vi "observacao.vi"() -> ()   [LabVIEW 2012]
uses:
  Control 1.ctl
  System.Windows.Forms
  Global_Telescopio.vi
  Global Tabs.vi
  Shared_160.lvlib
panel:
  out "timeStatShutterAlert":i32
  out "sendCommandShutter":bool
  out "shutterTimeOld":i32
  out "LEAF":i32
  in  "Default":string="DEFAULT"
  out "Flag ativo DEC":bool
  out "Flag ativo AH":bool
  out "Flag de erro p/ apagar lampada":bool
  out "Foco aux":dbl
  out "Cont-ShutOpen":timestamp
  out "Flag-ShutClose":bool
  out "Flag-ShutOpen":bool
  in  "erro lig":i32=3
  in  "erro des":i32=3
  in  "xxz":string
  out "Flag desligar":bool
  out "Flag ligar":bool
  out "Flag Stop":bool
  in  "AUX LAMPADA":bool
  out "Apontou":bool caption="Working Area"
  in  "AUX ABA":bool
  out "error out 5":errorcluster
  in  "error in (no error)":errorcluster
  out "AH_Destino":dbl format="%.9g"
  out "CONT DEC UTILS":i32
  out "CR DEC UTILS":i32
  out "CONT AH UTILS":i32
  out "CR AH UTILS":i32
  out "Erro PROTEC":i32=5
  out "Erro Lim":i32=5
  out "Flag Alarm":bool
  out "alarm Time":timestamp
  out "error out 4":errorcluster
  in  "Case Constant\n(See Context Help) 21":bool=TRUE
  in  "Case Constant\n(See Context Help) 20":bool=TRUE
  in  "Case Constant\n(See Context Help) 19":bool=TRUE
  in  "Case Constant\n(See Context Help) 18":bool
  in  "Case Constant\n(See Context Help) 17":bool=TRUE
  in  "Case Constant\n(See Context Help) 16":bool
  in  "LedPointing":bool=TRUE
  in  "Case Constant\n(See Context Help) 15":bool
  in  "Case Constant\n(See Context Help) 14":bool=TRUE
  in  "Case Constant\n(See Context Help) 13":bool=TRUE
  in  "Case Constant\n(See Context Help) 12":bool=TRUE
  in  "Case Constant\n(See Context Help) 11":bool
  in  "Case Constant\n(See Context Help) 10":bool
  in  "Case Constant\n(See Context Help) 9":bool
  in  "Disabled":u8=2
  in  "Case Constant\n(See Context Help) 8":bool=TRUE
  in  "Case Constant\n(See Context Help) 7":bool=TRUE
  in  "Case Constant\n(See Context Help) 6":bool
  in  "Case Constant\n(See Context Help) 5":bool
  in  "TRUE=HORA\nFALSE=GRAU":bool=TRUE
  in  "Case Constant\n(See Context Help) 4":bool
  in  "Case Constant\n(See Context Help) 3":bool
  in  "Case Constant\n(See Context Help) 2":bool
  in  "Case Constant\n(See Context Help)":bool
  out "TA3":u32
  out "TA2":u32
  out "TF2":u32
  out "TF1":u32
  out "TA1":u32
  out "Tick Cupula":u32
  out "T2 3":u32
  in  "ESTADO ABRIR":string
  in  "ESTADO FECHAR":string
  out "T2 2":u32
  out "T1 2":u32
  out "T2":u32
  out "T1":u32
  out "DEC":string="00 00 00,00"
  out "Hour Angle 2":string="00 00 0,00" caption="AH"
  in  "TIMER TICK":u32
  in  "STOP":bool
  in  "News":bool
  out "AtmosferaStr":string
  in  "BtShutterClose":bool caption="DOME SHUTTER"
  out "HA obs":dbl
  out "Time to Limit":string
  in  "Clear All Messages":bool
  out "FiltroDuplo":bool
  out "ObjCentrado":bool
  out "Timeout PROT":u32
  out "LIMITE":bool
  in  "DestCUP":i16
  in  "DestAH":dbl
  in  "DestDEC":dbl
  in  "M_CUP":i32
  out "TimeoutCUP 2":u32
  out "TimeoutAH 2":u32
  out "TimeoutDEC 2":u32
  in  "Max":dbl=2300.0
  in  "Min":dbl=200.0
  out "error out":errorcluster
  out "TUBO_STAT":string
  out "CUP_STAT":string
  out "DEC_STAT":string
  out "AH_STAT":string
  out "FOCO_ENC":string
  out "DEC_ENC":string
  out "AH_ENC":string
  out "RA on Target":bool
  in  "BtOnTatget":bool
  out "Offset DEC":dbl format="%#.2f"
  out "Offset RA":dbl format="%#.2f"
  out "Mount Fine Movement":bool
  out "Mount Gross Movement":bool
  in  "follow redirects (T)":bool=TRUE
  out "header":string
  out "subarray":string[][](array[string])
  out "Draw Area 4":cluster{"Width":u32, "Height":u32}
  out "Draw Area 3":cluster{"Width":u32, "Height":u32}
  in  "sair":bool
  out "Saida Path string":string
  out "AUX EDITA RA":string caption="Name"
  out "Sideral time":string caption="ST"
  out "UT":string
  out "FLAG SET COORD":bool
  out "AUX EDITA PMDEC":string caption="Name"
  out "AUX EDITA PMRA":string caption="Name"
  out "AUX EDITA EPOCH":string caption="Name"
  out "AUX EDITA DEC":string caption="Name"
  out "AUX EDITA Name":string caption="Name"
  out "Hour Angle":string="00 00 0,00"
  in  "DECTARGET":string
  in  "AHTARGET":string
  out "Zenital angle":dbl
  out "SlideEnviromental":dbl(slide) caption="Progress ..." scale=0.0..100.0
  out "RA AUX":string
  out "EPOCH AUX":string
  out "Draw Area 2":cluster{"Width":u32, "Height":u32}
  out "SYSTEM MESSAGES":string
  out "Data Acquisition Activity":bool
  out "Auto guider Activity":bool
  out "Security Zone":bool
  out "Precess Data out-of-date":bool
  out "D...":bool
  out "C...":bool
  out "B...":bool
  out "A...":bool
  out "DEC on Target":bool
  out "Dome on Target":bool
  out "Remote User in Control":bool
  out "Air Mass":dbl
  out "Epoch":dbl
  out "Right Ascention":string="00 00 00,00"
  out "Declination":string="00 00 00,00"
  out "Azimuth":dbl
  out "Wind Chill":dbl
  out "Boolean 11":bool
  out "Wind Dir":string
  in  "Int/Ext":bool=TRUE
  out "Temperature":dbl
  out "Humidity":dbl
  out "Dew Point":dbl
  out "Wind Speed":dbl
  out "Pressure":dbl
  in  "RESTART METEOR":bool
  in  "VARIABLE \nTRACKING":bool
  out "LED VAR TRACKING":bool
  out "LED GUIDER":bool
  out "Led Chave Dome":bool
  out "LED MOUNT":bool
  in  "GUIDER":bool
  in  "DOME":bool
  in  "MOUNT":bool
  out "NAME":string
  out "DEC":string
  out "RA":string
  in  "Tab Control":T1(tab)=enum."Test Only"
  in  "IMAGE 5":bool
  out "Image":picture
  in  "PictureBox":refnum<k24>(container)
  out "Image 2":picture
  in  "IMAGE 2":bool
  out "error out 3":errorcluster
  out "error out 2":errorcluster
  in  "IMAGE 4":bool
  out "Image 4":picture
  out "pressão atm":string
  out "hum local":string
  out "Temp amb":string
  in  "IMAGE 3":bool
  out "Image 3":picture
  in  "IMAGE 6":bool
  out "Image 3a":picture
  out "C. AH":i32
  out "DOMO_ENC":string
  out "Proteção":bool
  in  "M_PROT":i32
  out "dt":u32
  out "TUBO":bool[](array[boolean])
  out "CUP":bool[](array[boolean])
  out "DEC":bool[](array[boolean])
  out "RA":bool[](array[boolean])
  in  "statCUP":i32
  in  "statAH":i32
  in  "statDEC":i32
  out "statCUP 2":i32
  out "TimeoutCUP":u32
  out "Azimute cup":u16
  out "PosCUP":i16
  out "dtAUX2":u32
  out "dtAUX3":u32
  in  "Phx":dbl=200.0 caption="Setpoint" min=200.0 max=2300.0 step=1.0
  out "PosAH":dbl
  out "PosDEC":dbl
  out "dec=":bool
  out "ah=":bool
  in  "CR AH":i32
  in  "CR DEC":i32
  out "C. DEC":i32
  in  "M_AH":i32
  in  "M_DEC":i32
  in  "Stop All":bool
  in  "Setup, Pointing & Guiding":T2(tab)=enum."POINTING"
  in  "RA Max 2":i32 min=-6 max=23
  in  "RA Min 2":i32 min=-6 max=23
  out "Erro":bool
  in  "MAG Max":dbl min=-9.0 max=100.0
  in  "MAG Min":dbl min=-9.0 max=25.0
  in  "DEC Max":i32 min=-90 max=90
  in  "DEC Min":i32 min=-90 max=90
  in  "RA Max":i32 caption="AH Max" min=-6 max=23
  in  "RA Min":i32 caption="AH Min" min=-6 max=23
  in  "Filter RA":bool
  in  "Slide old":i32
  out "Tot Linhas":i32
  in  "Open BSC":bool
  in  "Slide":dbl(slide) min=0.0 max=24.0 step=0.024 scale format="%#_3g"
  in  "EDIT":bool
  in  "Insert":bool
  out "List File":string
  in  "Upload":bool
  in  "Open":bool
  in  "Save AS":bool
  in  "Save":bool
  in  "Clear ALL":bool
  in  "SET coord":bool
  in  "Delete":bool
  in  "Multicolumn Listbox":i32[](listbox)
  out "ScaleMin":string
  out "ScaleMax":string
  out "DEC obs":dbl format="%.9f"
  out "RA obs":dbl format="%.9f"
  in  "ChkPointPrecessed":bool
  in  "Processa Centragem":bool
  out "PM_DEC":string
  out "PM_RA":string
  out "LedPointing":bool caption="Telescope Pointing"
  out "TimeoutAH":u32
  out "TimeoutDEC":u32
  out "AtualDEC":dbl format="%.9f"
  out "MeanDEC":string
  out "MeanRA":string
  in  "MAG":string
  out "Zenital Angle":string
  out "Air Mass":string
  out "Tempo Obs":string
  in  "BtPointPrecess":bool
  in  "ChkCalGlobal":bool=TRUE
  in  "ChkCalLocal":bool caption="Use Local Zero"
  in  "ChkPoinLampOFF":bool=TRUE
  in  "ChkPointRNA":bool
  in  "ChkModel":bool=TRUE
  in  "ChkWindDown":bool
  in  "ChkOpenShutter":bool
  in  "ChkDomeEnable":bool
  out "LedPointWorkArea":bool caption="Working Area"
  in  "BtTargetPoint":bool
  out "StrPointTargetDEC":string caption="Declination"
  out "StrPointTargetRA":string caption="Right Ascension"
  in  "BtPointObjClear":bool
  in  "StrPointObjPMDEC":string caption="DEC Proper Motion"
  in  "StrPointObjPMRA":string caption="RA Proper Motion"
  in  "StrPointObjName":string caption="Name"
  in  "StrPointObjEpoch":string caption="Epoch"
  in  "StrPointObjDEC":string caption="Declination"
  in  "StrPointObjRA":string caption="Right Ascension"
  out "MOV_IDX_DEC":bool
  out "MOV_IDX_AH":bool
  out "LatchDeslocDEC":dbl caption="DEC"
  out "LatchDeslocRA":dbl caption="RA"
  in  "ClearDeslocDEC":bool
  in  "ClearDeslocRA":bool
  out "DeslocDEC":dbl caption="DEC" format="%#.1f"
  out "DeslocRA":dbl caption="RA" format="%#.1f"
  in  "Delete Calagem":bool
  in  "Global":bool caption="Local"
  in  "Calagem":bool
  in  "Up HS":bool
  in  "Right HS":bool
  in  "Down HS":bool
  in  "Left HS":bool
  in  "Velocity (arcsec/sec)":i32(slide) min=0 max=600 scale=0.0..600.0
  in  "BtPrecGO":bool
  in  "BtPrecCentrar":bool
  in  "PreciseOffsetDEC":dbl caption="DEC" min=-10000.0 max=10000.0 step=1.0 format="%.3g"
  in  "PreciseOffsetRA":dbl caption="RA . cos(delta)" min=-10000.0 max=10000.0 step=1.0 format="%.3g"
  in  "Habilita Movimento":bool=TRUE
  in  "Y STAR":i32=1 min=1 max=400 step=1
  in  "X STAR":i32=1 min=1 max=400 step=1
  in  "XY CENTER":bool
  in  "Y CENTER":i32=1 min=1 max=400 step=1
  in  "X CENTER":i32=1 min=1 max=400 step=1
  in  "ClearRA":bool
  in  "ClearDEC":bool
  in  "DEC RATE":i32 min=-2000 max=2000 step=1
  in  "RA  RATE":i32 min=-2000 max=2000 step=1
  out "x+y":timestamp
  in  "plus":bool
  in  "minus":bool
  in  "SetDefaultFocus":bool
  out "On Position":bool
  out "Foco":dbl(slide) scale=200.0..2300.0
  in  "Setpoint":dbl=200.0 min=200.0 max=2300.0 step=1.0
  in  "GO":bool
  in  "Focus +":bool
  in  "Focus -":bool
  in  "New Angle":string="    0.0"
  out "Default Angle":string="      0.00"
  in  "SetRotatorDefAngle":bool
  in  "Set Rotator Angle":bool
  out "Rotator Angle":string="  0.00" caption="for  GUIDING"
  out "StatShutterFile":string
  out "Command":string
  in  "CCW":bool
  out "RefreshShutterState":bool
  in  "BtParavStop":bool
  in  "BtParavUp":bool
  in  "BtParavDown":bool
  out "LedShutter":bool
  out "TimeoutTrap":u32
  out "StatShutter":string caption="Control State"
  in  "BtShutClose":bool
  in  "BtShutOpen":bool
  out "StatDome":string caption="Control State"
  in  "BtDomeSTOP":bool
  in  "BtDomeGO":bool caption="DOME"
  in  "DomeNewPos":i32=30 caption="New Position" min=0 max=360
  out "PosCup":i16 caption="Position"
  in  "CW":bool
  out "LED ACTION":bool
  out "LED MODE":bool
  in  "ACTION":bool
  in  "MODE":bool
  in  "Default Met":bool=TRUE
  in  "PROTEÇÃO":bool
  in  "STOP":bool
  in  "Enable Centragem":bool=TRUE
  in  "GO":bool
  in  "StrPointObjDEC 2":string caption="DEC"
  in  "StrPointObjRA 2":string caption="AH"
  out "MOVING":bool
  in  "FLAT-FIELD":bool
  in  "BtUtilPark":bool
  in  "ECASS":bool
  in  "BtUtilZenith":bool
  in  "TabInstrumento":T3(tab)=enum."Cam 1"
  out "Posição Rede":i32=10 caption="Largura da Fenda" min=10 max=5000 step=1
  in  "HomePrisma":T4 caption="DOME"
  in  "HomeEspelho":T4 caption="DOME"
  in  "HomeFenda":T4 caption="DOME"
  in  "IronArc":bool=TRUE
  out "Boolean":bool
  out "Largura da Fenda 2":dbl=10.0 caption="Largura da Fenda" min=10.0 max=5000.0 step=1.0
  in  "Prisma das Lâmpadas":bool
  out "Position":string
  in  "Largura da Fenda":dbl=10.0 min=10.0 max=5000.0 step=1.0
  in  "Go Largura da Fenda":bool caption="DOME"
  in  "Angulo da rede de difração":i32=10 caption="Ângulo da Rede" min=10 max=99989 step=1
  in  "Go Angulo de Difração":bool caption="DOME"
  in  "Incand":bool=TRUE
  in  "Neon":bool=TRUE
  in  "Cathode":bool=TRUE
  out "Ang. Fenda":dbl
  in  "Go_Coudé":bool
  in  "Radio Buttons":enum32{"Azul", "Visível", "Vermelho"}(radio)
  out "EndTime":u32
  out "ledAzul":bool
  out "ledVisivel":bool
  out "ledVermelho":bool
  in  "MENSAGEM":string="EM MOVIMENTO"
  out "MENSAGEM 2":string="EM MOVIMENTO"
  out "#2":bool
  out "#3":bool
  out "#4":bool
  out "PosSecundario":bool
  out "Cjto_3":bool
  out "EspAtual":string
  out "parou":bool
  out "parou 2":bool
  out "Posição Espelho":dbl=10.0 caption="Largura da Fenda" min=10.0 max=5000.0 step=1.0
  out "parou 3":bool
  out "Output Message":string
  in  "stopEcass":bool
  out "SlideEcass":u8(slide) caption="Espelho movendo..." max=100 scale=0.0..100.0
  out "LedRep":bool
  out "LedCal":bool
  in  "Sent_EspLampCass":bool
  out "LedHe":bool
  out "LedNe":bool
  in  "He-Ar":bool
  in  "Ne":bool
  in  "stopCam1":bool
  out "SlideCam1":u8(slide) caption="Espelho movendo..." max=100 scale=0.0..100.0
  out "LedRepCam1":bool
  out "LedCalCam1":bool
  in  "Sent_EspDesvFeixe":bool
  in  "Go_filtro":bool
  in  "Filtro":string(combo)
  in  "Mover/Parar":bool
  out "Recuar":bool
  in  "Sentido":bool=TRUE
  in  "Velocidade":bool
  out "Rapido":bool
  out "Lento":bool
  out "Avancar":bool
  out "Comando":string
  in  "Mensage Alarme":string="To light up close the Shutter !"
  out "CoudeSel":bool
  in  "Coude":bool
  in  "BtCalFlatField":bool
  in  "ChkCalLamp4":bool
  in  "ChkCalLamp3":bool
  in  "ChkCalLamp2":bool
  in  "ChkCalLamp1":bool
  in  "BtCalTurnOff":bool
  in  "BtCalTurnOn":bool
  out "StrongSel":bool
  out "MediumSel":bool
  out "WeakSel":bool
  in  "Strong":bool
  in  "Medium":bool
  in  "Weak":bool
  # "TELESCOPE CONTROL SYSTEM\nPICO DOS DIAS OBSERVATORY"
  # "Status Information"
  # "System Positions"
  # "Environmental Status"
  # "EXT"
  # "INT"
  # "mBar"
  # "o"
  # "C"
  # "Km/h"
  # "%"
  # "o"
  # "o"
  # "C"
  # "C"
  # "CLOUSURE LIMITS"
  # "Wind Speed            >  70 Km/h\nRelative Humidity    >  97 %\nInternal Dewpoint  <  0.5  C\nExternal Dewpoint <  1.0  C"
  # "OBJECT"
  # "TRACKING ENABLE"
  # "Conector 4"
  # "Conector 3"
  # "ALARME\nATENÇÃO\nERROS\nOCUPADO"
  # "Proteção\n\nTracking\nVar_Track"
  # "Rapido\nLigeiro\nFino\nRun"
  # "Motor\nIDX_Rdy\nManual"
  # "BSC FILTERS"
  # "LIST FILE"
  # "OBJECT INPUT"
  # "TARGET"
  # "OPTIONS"
  # "MANUAL OFFSET"
  # "PRECISE OFFSET"
  # "N"
  # "E"
  # "W"
  # "arcsec"
  # "arcsec"
  # "S"
  # "DISPLACEMENT"
  # "CALAGEM"
  # "PODE NÃO FUNCIONAR CORRETAMENTE!"
  # "STAR CENTERING"
  # "VAR. TRACKING"
  # "AUTO-GUIDER COORDINATES"
  # "1) Entrar X e Y do cursor do Autoguider correspondente à posição de centragem nas entradas X CENTER e Y CENTER. \n2) Após apontamento, entrar em X STAR e Y STAR os valores de X e Y do Autoguider com o \"Guide Box\" sobre o objeto apontado. \n3) Clicar em MOVE STAR TO CENTER."
  # "Focus Position"
  # "(instrument)"
  # "Continuous Movement"
  # "Fine Tuning"
  # "ATENÇÃO:\nO Rotator ainda não está integrado ao sistema de controle e como sua posição afeta a guiagem, sempre que o rotator for girado manualmente é necessário digitar o valor de sua nova posição no controle \"New Angle\" e pressionar \"SET NEW\".\n\nPressionar \"SET NEW\" ou \"SET DEFAULT\" não gira o rotator!"
  # "ROTATION"
  # "SHUTTER"
  # "WINDSCREEN"
  # "Covers"
  # "FIXED POSITIONS"
  # "Acquisition System\nON TARGET command"
  # "Select one Mirrror"
  # "Mirror #2"
  # "Mirror #3"
  # "Mirrors Drivers"
  # "Lâmpadas de Calibração"
  # "Espelho das Lâmpadas de Calibração"
  # "Posição"
  # "Repouso"
  # "Ativo"
  # "LIGA"
  # "LIGA"
  # "DESL."
  # "DESL."
  # "Espelho do Eucalyptus"
  # "Roda de filtros"
  # "Posição"
  # "Repouso"
  # "Ativo"
  # "Espelho de Campo"
  # "Recuar"
  # "Avançar"
  # "Rápido"
  # "Lento"
  # "CALIBRATION LAMPS"
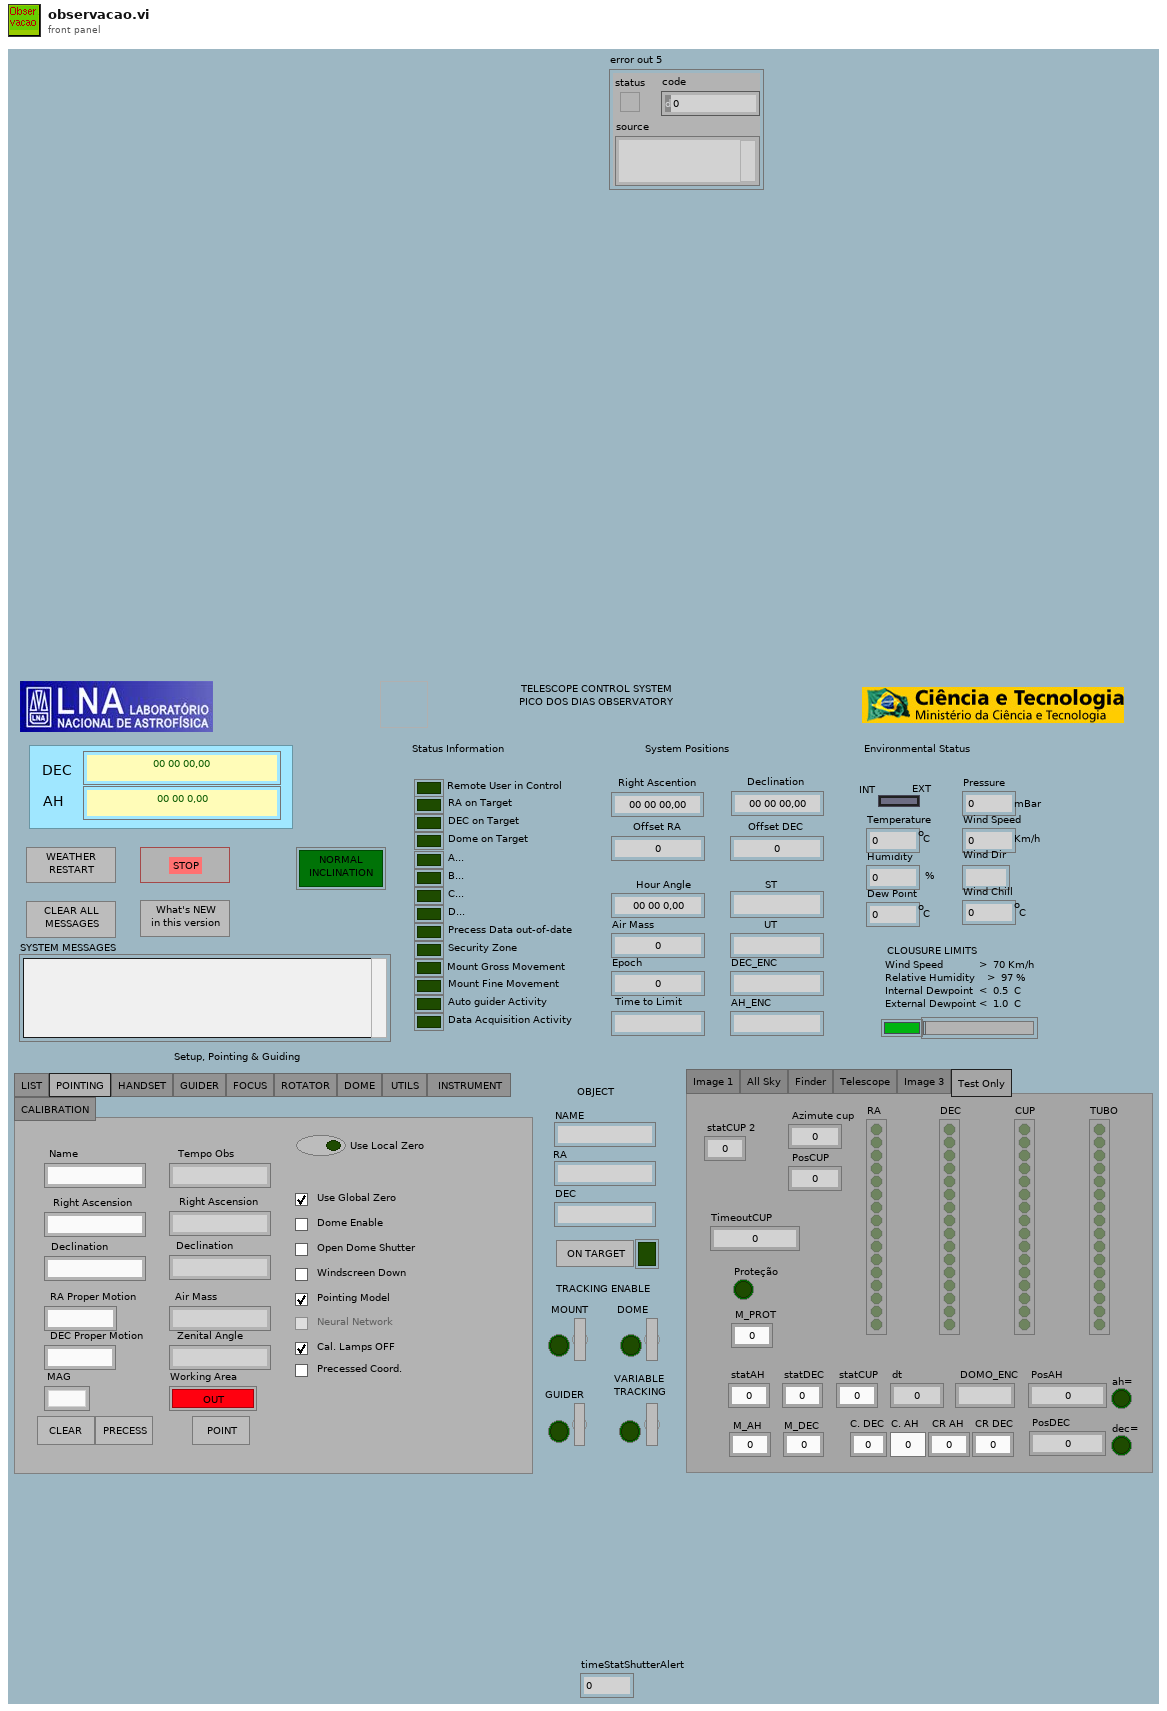
[diagram p1: front panel]
types:
  T1 = enum32{"Image 1", "All Sky", "Finder", "Telescope", "Image 3", "Test Only"}
  T2 = enum32{"LIST", "POINTING", "HANDSET", "GUIDER", "FOCUS", "ROTATOR", "DOME", "UTILS ", " INSTRUMENT ", "CALIBRATION"}
  T3 = enum32{"Coude", "Casseg.", "Eucalyp.", "Cam 1", "Cam 2", "Cam IV.", "Polarim.", "Fotrap"}
  T4 = typedef "Control 1.ctl" = bool
  T5 = enum32{"Page Enabled", "Page Disabled", "Page Disabled & Grayed"}
  T6 = enum16{"open", "replace", "create", "open or create", "replace or create", "replace or create with confirmation"}
  T7 = enum16{"open", "open or create", "create or replace", "create"}
  T8 = enum16{"open", "open or create", "create or replace", "create", "open (read only)"}
  T9 = typedef "LVRemotePanelConnectionsTypeDef.ctl" = cluster{"VI Name":string, "Remote":string, "UserName":string, "Port":i32, "Status":enum32{"Viewing", "Waiting For Control", "Controlling"}, "Create Time":timestamp, "Status Time":timestamp, "Control End Time":timestamp}[]
  T10 = enum8{"Enabled", "Disabled", "Disabled and Grayed Out"}
  T11 = cluster{"left":i16, "top":i16, "right":i16, "bottom":i16}
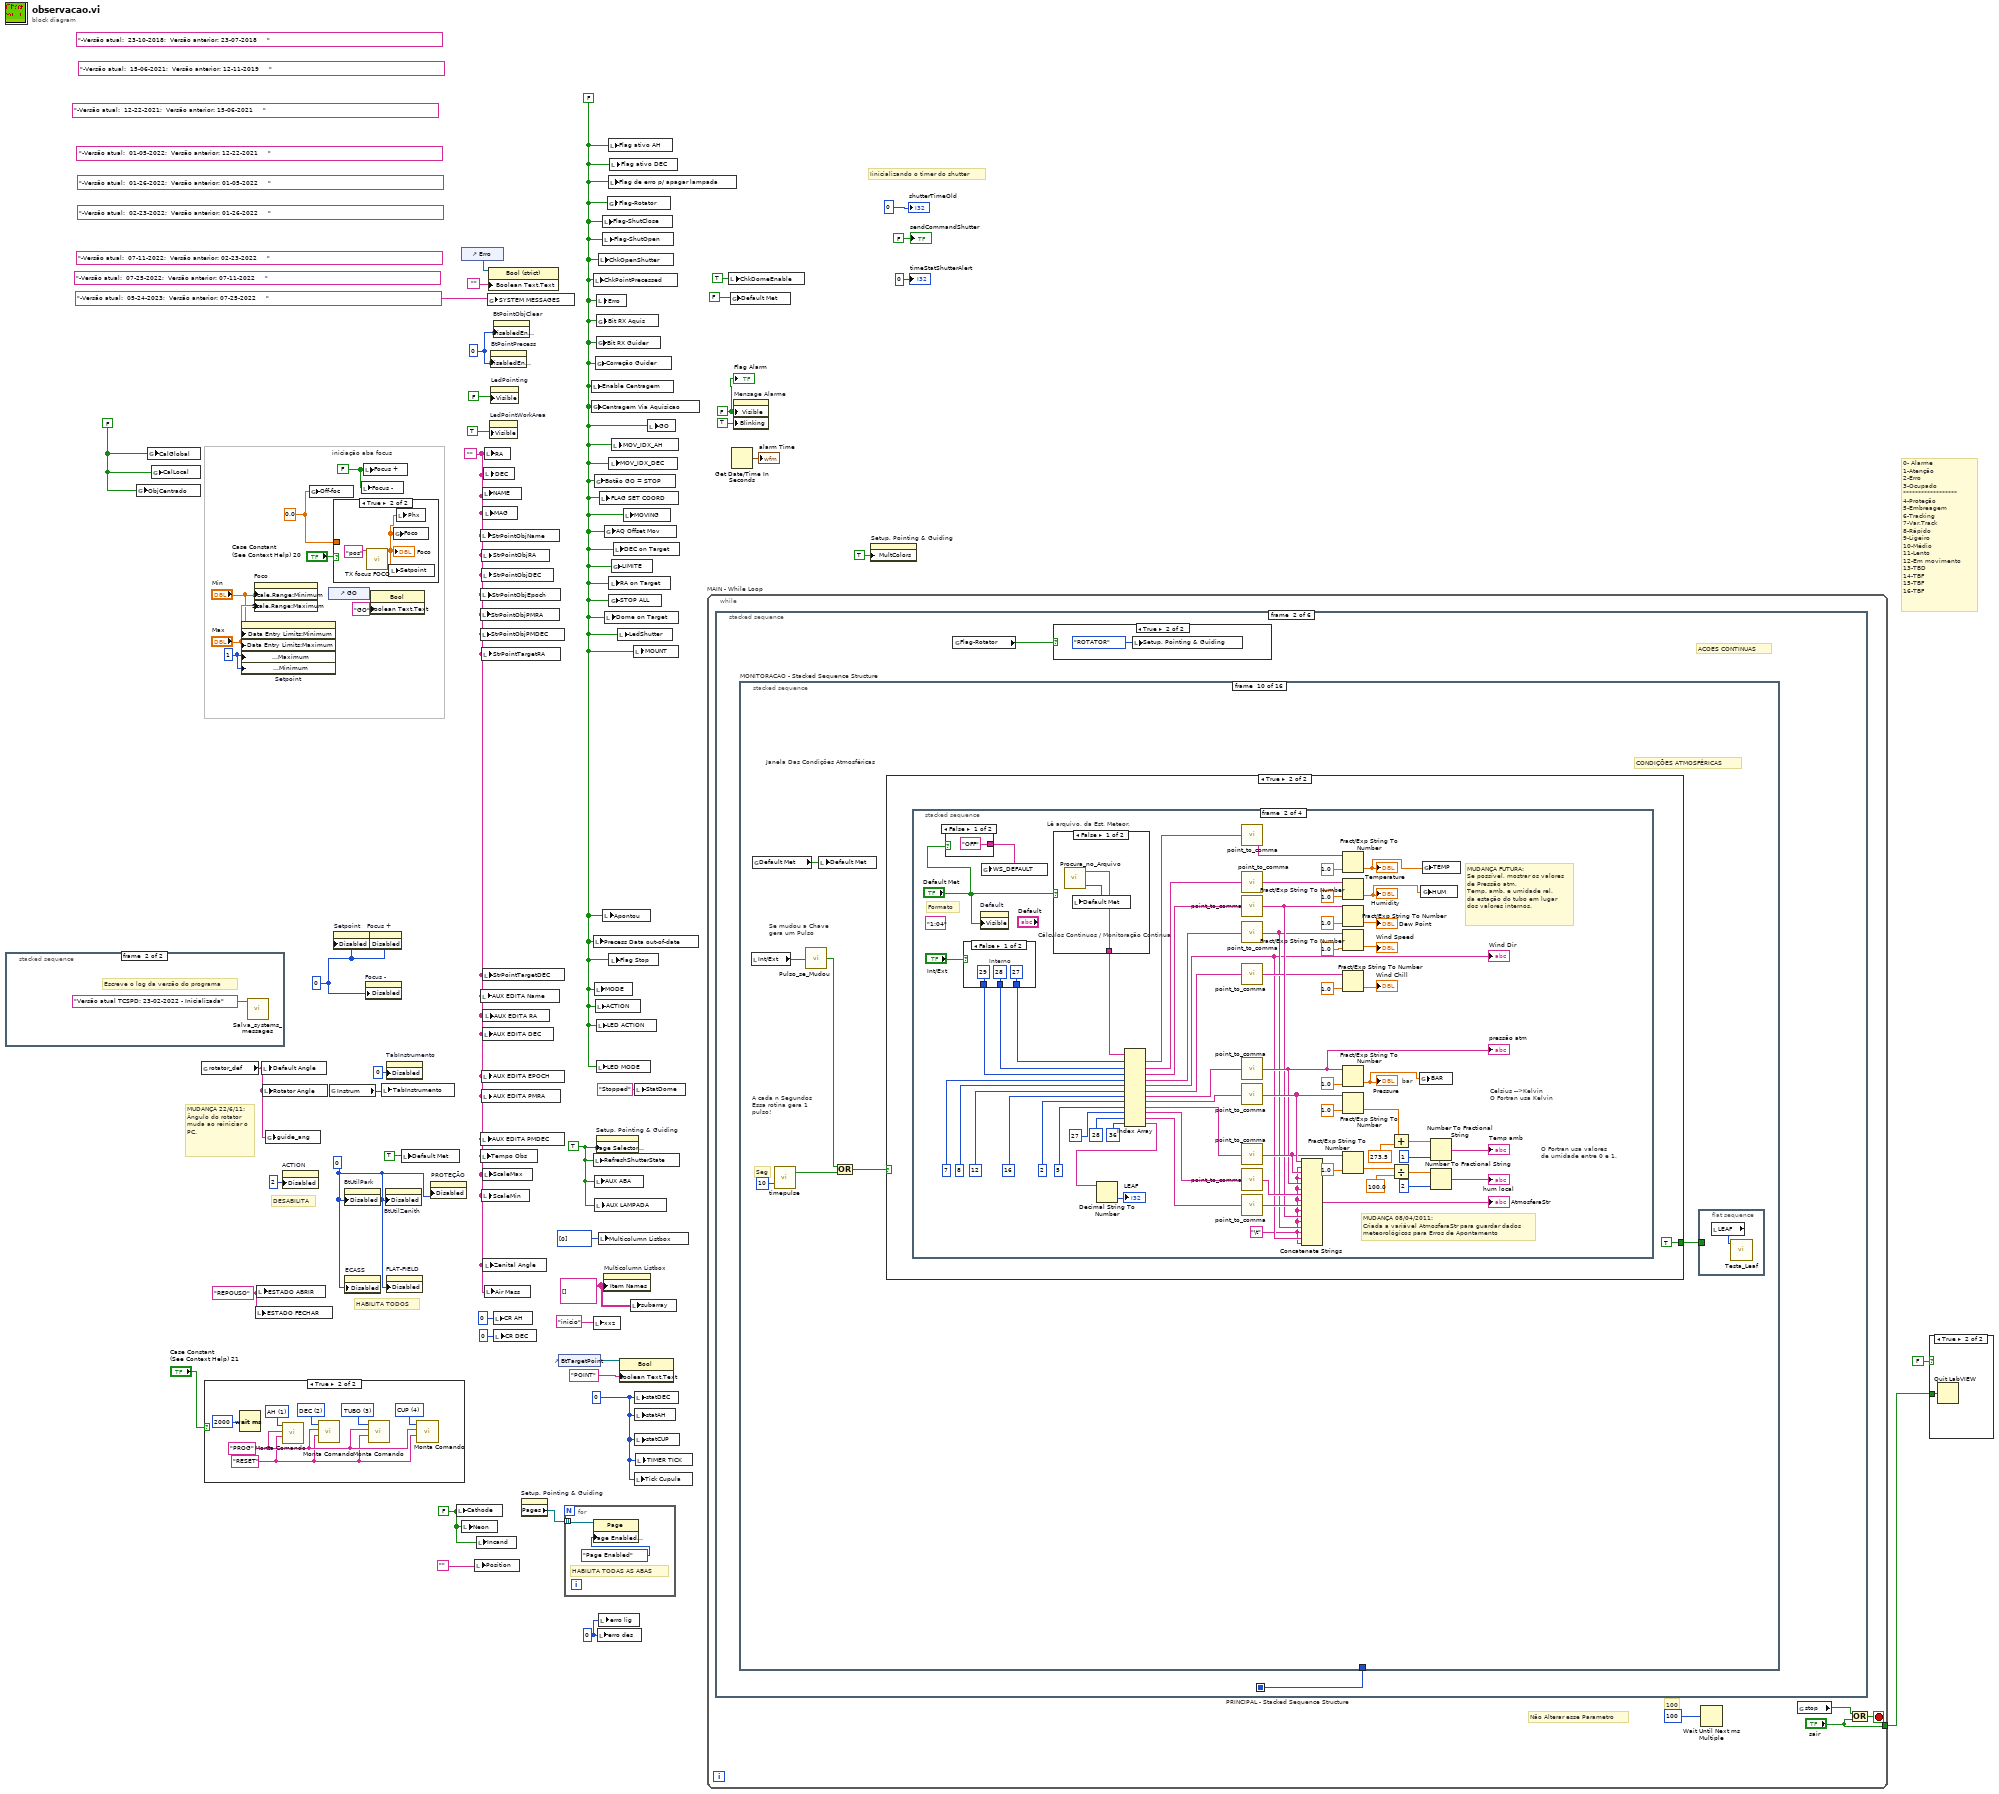
[diagram p0: block diagram]
diagram:
  (unwired) "-Versão atual:  07-25-2022;  Versão anterior: 07-11-2022     " ("SYSTEM MESSAGES")
  (unwired) "-Versão atual:  07-11-2022;  Versão anterior: 02-23-2022     " ("SYSTEM MESSAGES")
  (unwired) "-Versão atual:  02-23-2022;  Versão anterior: 01-26-2022     " ("SYSTEM MESSAGES")
  (unwired) "-Versão atual:  01-26-2022;  Versão anterior: 01-05-2022     " ("SYSTEM MESSAGES")
  (unwired) "-Versão atual:  01-05-2022;  Versão anterior: 12-22-2021     " ("SYSTEM MESSAGES")
  (unwired) "-Versão atual:  12-22-2021;  Versão anterior: 15-06-2021     " ("SYSTEM MESSAGES")
  (unwired) "-Versão atual:  15-06-2021;  Versão anterior: 12-11-2019     " ("SYSTEM MESSAGES")
  w9 = 0
  w10 = 0 ("erro des")
  w16 = FALSE ("Visible")
  w20 = FALSE ("ThAr")
  w22 = "REPOUSO" ("y")
  (unwired) "-Versão atual:  23-10-2018;  Versão anterior: 23-07-2018     " ("SYSTEM MESSAGES")
  w34 = u8 0 ("Disabled")
  w12 = TRUE ("Page Selector Visible")
  w37 = u8 1 ("OutOfRngActMin")
  w40 = FALSE ("Set aux")
  w41 = u8 0 ("Disabled")
  w42 = FALSE ("Set aux")
  w43 = 0.0 ("Offset")
  w21 = 0 ("estado")
  w29 = ""
  w48 = string[][] [] ("Item Names")
  w8 = FALSE ("Set aux")
  # "Iinicializando o timer do shutter"
  # "DESABILITA"
  # "MUDANÇA 22/6/11:\nÂngulo do rotator muda ao reiniciar o PC."
  # "HABILITA TODOS"
  # "0- Alarme\n1-Atenção\n2-Erro\n3-Ocupado\n******************\n4-Proteção\n5-Embreagem\n6-Tracking\n7-Var.Track\n8-Rápido\n9-Ligeiro\n10-Médio\n11-Lento\n12-Em movimento\n13-TBD\n14-TBF\n15-TBF\n16-TBF"
  # "iniciação aba focus"
  n1 = stacked-sequence {
    frame #0 {
      # "Escreve o log da estação\nmetereologica"
      # "Alterado 11/12/2012 est.\nmeteorológica"
      n2 = call "Teste_Read_Meteorologica.vi"() -> ()  [unwired: 2 in, 1 out]
    }
    frame #1 {
      # "Escreve o log da versão do programa"
      n3 = call "Salva_systems_messages.vi"("Mensagem"="Versão atual TCSPD: 23-02-2022 - Inicializada" ("message")) -> ()  [unwired: 5 in]
    }
  }
  n4 = global write "Global_Telescopio.vi" "ObjCentrado"(w40) -> ()
  n5 = global write "Global_Telescopio.vi" "CalGlobal"(w40) -> ()
  n6 = global write "Global_Telescopio.vi" "CalLocal"(w40) -> ()
  n7 = global read "Global_Telescopio.vi" "rotator_def"() -> (w25:string)
  n8 = case shown="True" "Case Constant\n(See Context Help) 21" {
    frame False {
    }
    frame True {
      w55 = u16 4 items=["ZERO", "AH", "DEC", "TUBO", "CUP"] ("Controlador")
      w56 = u16 3 items=["ZERO", "AH", "DEC", "TUBO", "CUP"] ("Controlador")
      w58 = u16 2 items=["ZERO", "AH", "DEC", "TUBO", "CUP"] ("Controlador")
      w54 = "PROG" ("Comando")
      w53 = "RESET" ("Comando")
      w59 = u16 1 items=["ZERO", "AH", "DEC", "TUBO", "CUP"] ("Controlador")
      n9 = Wait (ms)(milliseconds to wait=u32 2000) -> ()  [unwired: 1 out]
      n10 = call "Monta Comando.vi"("Comando"=w53, "Dispositivo"=w54, "Controlador"=w59) -> ()  [unwired: 4 in, 3 out]
      n11 = call "Monta Comando.vi"("Comando"=w53, "Dispositivo"=w54, "Controlador"=w58) -> ()  [unwired: 4 in, 3 out]
      n12 = call "Monta Comando.vi"("Comando"=w53, "Dispositivo"=w54, "Controlador"=w56) -> ()  [unwired: 4 in, 3 out]
      n13 = call "Monta Comando.vi"("Comando"=w53, "Dispositivo"=w54, "Controlador"=w55) -> ()  [unwired: 4 in, 3 out]
    }
  }
  n14 = property on="Setpoint" class="DigNum (strict)"("Data Entry Limits:Minimum"="Min", "Data Entry Limits:Maximum"="Max", "Response to Value Outside Limits:Maximum"=w37, "Response to Value Outside Limits:Minimum"=w37) -> ()  [unwired: 2 in, 2 out]
  n15 = property on="Foco" class="Slide (strict)"("Scale.Range:Minimum"="Min", "Scale.Range:Maximum"="Max") -> ()  [unwired: 2 in, 2 out]
  n16 = local write "ESTADO FECHAR"(w22) -> ()
  n17 = local write "ESTADO ABRIR"(w22) -> ()
  n18 = local write "Default Angle"(w25) -> ()
  n19 = local write "Rotator Angle"(w25) -> ()
  n20 = global write "Global_Telescopio.vi" "guide_ang"(w25) -> ()
  n21 = property on="ACTION" class="Bool (strict)"("Disabled"=u8 2) -> ()  [unwired: 2 in, 2 out]
  n22 = global write "Global Tabs.vi" "Off-foc"(w43) -> ()
  n23 = control-ref of="GO"() -> (w46:refnum<vi>)
  n24 = global read "Global_Telescopio.vi" "Instrum"() -> (w32:u16)
  n25 = property on="Setpoint" class="DigNum (strict)"("Disabled"=w41) -> ()  [unwired: 2 in, 2 out]
  n26 = case shown="True" "Case Constant\n(See Context Help) 20" {
    tunnel: w43 -> [_ _]
    frame False {
    }
    frame True {
      n27 = call "TX focus FOCO.vi"("Comando"="pos") -> ("pos (deg)"=w60:dbl)  [unwired: 12 in, 2 out]
      "Foco" <- w60
      n28 = local write "Setpoint"(w60) -> ()
      n29 = global write "Global_Telescopio.vi" "Foco"(w60) -> ()
      n30 = local write "Phx"(w60) -> ()
    }
  }
  n31 = property on="BtUtilPark" class="Bool (strict)"("Disabled"=w34) -> ()  [unwired: 2 in, 2 out]
  n32 = property on="ECASS" class="Bool (strict)"("Disabled"=w34) -> ()  [unwired: 2 in, 2 out]
  n33 = local write "Focus -"(w42) -> ()
  n34 = local write "Focus +"(w42) -> ()
  n35 = property on="Focus +" class="Bool (strict)"("Disabled"=w41) -> ()  [unwired: 2 in, 2 out]
  n36 = property on="Focus -" class="Bool (strict)"("Disabled"=w41) -> ()  [unwired: 2 in, 2 out]
  n37 = property class="Bool"(reference=w46, "Boolean Text.Text"="GO") -> ()  [unwired: 1 in, 2 out]
  n38 = local write "TabInstrumento"(w32) -> ()
  n39 = property on="BtUtilZenith" class="Bool (strict)"("Disabled"=w34) -> ()  [unwired: 2 in, 2 out]
  n40 = property on="TabInstrumento" class="TabCtl (strict)"("Disabled"=u8 0) -> ()  [unwired: 2 in, 2 out]
  n41 = property on="FLAT-FIELD" class="Bool (strict)"("Disabled"=w34) -> ()  [unwired: 2 in, 2 out]
  n42 = local write "Default Met"(TRUE ("Default Met")) -> ()
  n43 = property on="PROTEÇÃO" class="Bool (strict)"("Disabled"=w34) -> ()  [unwired: 2 in, 2 out]
  n44 = local write "Cathode"(w20) -> ()
  n45 = control-ref of="Erro"() -> (w30:refnum<vi>)
  n46 = local write "Neon"(w20) -> ()
  n47 = local write "Position"("") -> ()
  n48 = local write "Incand"(w20) -> ()
  n49 = local write "StrPointObjPMRA"(w29) -> ()
  n50 = local write "StrPointObjPMDEC"(w29) -> ()
  n51 = local write "Tempo Obs"(w29) -> ()
  n52 = local write "StrPointObjName"(w29) -> ()
  n53 = local write "StrPointObjEpoch"(w29) -> ()
  n54 = local write "AUX EDITA Name"(w29) -> ()
  n55 = local write "AUX EDITA PMDEC"(w29) -> ()
  n56 = local write "StrPointObjRA"(w29) -> ()
  n57 = local write "StrPointObjDEC"(w29) -> ()
  n58 = local write "StrPointTargetRA"(w29) -> ()
  n59 = local write "AUX EDITA EPOCH"(w29) -> ()
  n60 = local write "AUX EDITA PMRA"(w29) -> ()
  n61 = local write "ScaleMin"(w29) -> ()
  n62 = local write "NAME"(w29) -> ()
  n63 = local write "StrPointTargetDEC"(w29) -> ()
  n64 = local write "AUX EDITA DEC"(w29) -> ()
  n65 = local write "ScaleMax"(w29) -> ()
  n66 = local write "MAG"(w29) -> ()
  n67 = local write "AUX EDITA RA"(w29) -> ()
  n68 = local write "Zenital Angle"(w29) -> ()
  n69 = local write "DEC"(w29) -> ()
  n70 = local write "RA"(w29) -> ()
  n71 = local write "Air Mass"(w29) -> ()
  n72 = global write "Global_Telescopio.vi" "SYSTEM MESSAGES"("-Versão atual:  05-24-2023;  Versão anterior: 07-25-2022     " ("SYSTEM MESSAGES")) -> ()
  n73 = property class="Bool (strict)"(reference=w30, "Boolean Text.Text"="") -> ()  [unwired: 1 in, 2 out]
  n74 = property on="LedPointWorkArea" class="Bool (strict)"("Visible"=TRUE ("GUIDING")) -> ()  [unwired: 2 in, 2 out]
  n75 = property on="BtPointPrecess" class="Bool"("DisabledEnum"=w9) -> ()  [unwired: 2 in, 2 out]
  n76 = property on="LedPointing" class="Bool (strict)"("Visible"=FALSE ("Set aux")) -> ()  [unwired: 2 in, 2 out]
  n77 = property on="BtPointObjClear" class="Bool"("DisabledEnum"=w9) -> ()  [unwired: 2 in, 2 out]
  n78 = local write "CR AH"(0 ("CR AH")) -> ()
  n79 = local write "CR DEC"(0 ("CR DEC")) -> ()
  n80 = property on="Setup, Pointing & Guiding" class="TabCtl (strict)"() -> ("Pages"=w35:refnum<vi>[])  [unwired: 2 in, 2 out]
  n81 = control-ref of="BtTargetPoint"() -> (w50:refnum<vi>)
  n82 = for {
    tunnel: w35 -> [w63] mode=indexing
    # "HABILITA TODAS AS ABAS"
    n83 = property class="Page"(reference=w63, "Page Enabled State"=T5."Page Enabled") -> ()  [unwired: 1 in, 2 out]
  }
  n84 = local write "Enable Centragem"(w8) -> ()
  n85 = global write "Global_Telescopio.vi" "Centragem Via Aquisicao"(w8) -> ()
  n86 = local write "ChkPointPrecessed"(w8) -> ()
  n87 = local write "Precess Data out-of-date"(w8) -> ()
  n88 = local write "RefreshShutterState"(w12) -> ()
  n89 = local write "xxz"("inicio") -> ()
  n90 = global write "Global_Telescopio.vi" "Botão GO = STOP"(w8) -> ()
  n91 = local write "MODE"(w8) -> ()
  n92 = local write "AUX ABA"(w12) -> ()
  n93 = local write "AUX LAMPADA"(w12) -> ()
  n94 = global write "Global_Telescopio.vi" "Correção Guider"(w8) -> ()
  n95 = local write "ACTION"(w8) -> ()
  n96 = global write "Global_Telescopio.vi" "Bit RX Guider"(w8) -> ()
  n97 = local write "LED ACTION"(w8) -> ()
  n98 = local write "LED MODE"(w8) -> ()
  n99 = property on="Setup, Pointing & Guiding" class="TabCtl (strict)"("Page Selector Visible"=w12) -> ()  [unwired: 2 in, 2 out]
  n100 = local write "Erro"(w8) -> ()
  n101 = global write "Global_Telescopio.vi" "Bit RX Aquis"(w8) -> ()
  n102 = local write "erro des"(w10) -> ()
  n103 = local write "ChkOpenShutter"(w8) -> ()
  n104 = local write "Multicolumn Listbox"(i32[] [0] ("Multicolumn Listbox")) -> ()
  n105 = local write "erro lig"(w10) -> ()
  n106 = local write "FLAG SET COORD"(w8) -> ()
  n107 = local write "Flag-ShutClose"(w8) -> ()
  n108 = local write "Flag-ShutOpen"(w8) -> ()
  n109 = local write "Apontou"(w8) -> ()
  n110 = property on="Multicolumn Listbox" class="MCListbox (strict)"("Item Names"=w48) -> ()  [unwired: 2 in, 2 out]
  n111 = global write "Global_Telescopio.vi" "AQ Offset Mov"(w8) -> ()
  n112 = local write "Dome on Target"(w8) -> ()
  n113 = global write "Global_Telescopio.vi" "Flag-Rotator"(w8) -> ()
  n114 = local write "Flag ativo AH"(w8) -> ()
  n115 = local write "Flag de erro p/ apagar lampada"(w8) -> ()
  n116 = local write "MOV_IDX_DEC"(w8) -> ()
  n117 = local write "RA on Target"(w8) -> ()
  n118 = global write "Global_Telescopio.vi" "STOP ALL"(w8) -> ()
  n119 = local write "Flag Stop"(w8) -> ()
  n120 = local write "Flag ativo DEC"(w8) -> ()
  n121 = global write "Global_Telescopio.vi" "LIMITE"(w8) -> ()
  n122 = local write "MOV_IDX_AH"(w8) -> ()
  n123 = local write "DEC on Target"(w8) -> ()
  n124 = local write "LedShutter"(w8) -> ()
  n125 = property class="Bool"(reference=w50, "Boolean Text.Text"="POINT") -> ()  [unwired: 1 in, 2 out]
  n126 = local write "MOVING"(w8) -> ()
  n127 = local write "subarray"(w48) -> ()
  n128 = local write "MOUNT"(w8) -> ()
  n129 = local write "Tick Cupula"(w21) -> ()
  n130 = local write "StatDome"("Stopped" ("Status")) -> ()
  n131 = local write "statDEC"(w21) -> ()
  n132 = local write "statAH"(w21) -> ()
  n133 = local write "statCUP"(w21) -> ()
  n134 = local write "TIMER TICK"(w21) -> ()
  n135 = local write "GO"(w8) -> ()
  n136 = while "MAIN - While Loop" {
    tunnel: ["sair"] -> w47
    stop <- w66 stop-if-true
    # "100"
    # "Não Alterar esse Parametro"
    n137 = stacked-sequence "PRINCIPAL - Stacked Sequence Structure" {
      seq-local: [w71 _ _ _ _ _] -> [_ w74 _ _ _ w4089]
      frame #0 {
        # "CLIENTE REMOTO"
        # "Verifica se Existe Cliente Remoto Conectado"
        n138 = invoke class="VI" method="RP.Client Connections"() -> ("Connections"=w72:T9, "Controller"=w70:i32)  [unwired: 5 in, 3 out]
        n139 = Equal?(x=w70, y=0) -> (x = y?=→"Remote User in Control":bool)
        n140 = global write "Global_Telescopio.vi" "Controller Rem/Loc"(w70) -> ()
        n141 = global write "Global_Telescopio.vi" "Dados do Computador Remoto Conectado"(w72) -> ()
        n142 = Tick Count (ms)() -> (millisecond timer value=w71:u32)
      }
      frame #1 {
        # "ACOES CONTINUAS"
        # "Cálculos Continuos / Monitoração Continua"
        n143 = stacked-sequence "MONITORACAO - Stacked Sequence Structure" {
          tunnel: w74 -> [_ _ _ w447 _ _ _ _ _ _ _ _ _ _ _ _]
          frame #0 {
            w106 = u16 3 items=["ZERO", "AH", "DEC", "TUBO", "CUP", "CASS", "COUDE"] ("Controlador")
            w114 = u16 4 items=["ZERO", "AH", "DEC", "TUBO", "CUP", "CASS", "COUDE"] ("Controlador")
            w115 = u16 2 items=["ZERO", "AH", "DEC", "TUBO", "CUP", "CASS", "COUDE"] ("Controlador")
            w118 = u16 1 items=["ZERO", "AH", "DEC", "TUBO", "CUP", "CASS", "COUDE"] ("Controlador")
            # "Monitora o programa para enviar comando\ntrapeira parar após 40s"
            # "Grava o valor do foco \natual a cada minuto"
            # "PROCESSO LE ENCODERS"
            # "Colocar neste frame a leitura de status dos outros controladores"
            # "LEITURA STATUS DOS CONTROLADORES"
            n144 = Get Date/Time In Seconds() -> (seconds since 1Jan1904=w86:timestamp)
            n145 = Format Date/Time String(time format string (%c)="%S", seconds (now)=w86) -> (date/time string=w85:string)  [unwired: 1 in]
            n146 = case shown="False" "Case Constant\n(See Context Help)" {
              selector: "Case Constant\n(See Context Help)" -> [_ w210]
              tunnel: [w209 w210] -> w116
              tunnel: w115 -> [w208 _]
              tunnel: [w207 _] -> w117
              tunnel: [w206 _] -> w88
              tunnel: [w205 _] -> w101
              frame False {
                n147 = call "Get Status Controlador.vi"("Controlador"=w208) -> ("Status"=w205:string, "Parametros"=w207:string, "Bits Status"=w206:bool[], "Erro comunicação"=w209:bool)
              }
              frame True {
              }
            }
            "DEC_STAT" <- w101
            "DEC" <- w88
            n148 = case shown="False" "Case Constant\n(See Context Help)" {
              selector: "Case Constant\n(See Context Help)" -> [_ w204]
              tunnel: [w203 w204] -> w113
              tunnel: w114 -> [w202 _]
              tunnel: [w201 _] -> w112
              tunnel: [w200 _] -> w98
              tunnel: [w199 _] -> w100
              frame False {
                n149 = call "Get Status Controlador.vi"("Controlador"=w202) -> ("Status"=w199:string, "Parametros"=w201:string, "Bits Status"=w200:bool[], "Erro comunicação"=w203:bool)
              }
              frame True {
              }
            }
            "CUP_STAT" <- w100
            "CUP" <- w98
            n150 = case shown="False" "Case Constant\n(See Context Help)" {
              selector: "Case Constant\n(See Context Help)" -> [_ w194]
              tunnel: [w193 w194] -> w107
              tunnel: w106 -> [w192 _]
              tunnel: [w191 _] -> w108
              tunnel: [w190 _] -> w96
              tunnel: [w189 _] -> w99
              frame False {
                n151 = call "Get Status Controlador.vi"("Controlador"=w192) -> ("Status"=w189:string, "Parametros"=w191:string, "Bits Status"=w190:bool[], "Erro comunicação"=w193:bool)
              }
              frame True {
              }
            }
            "TUBO_STAT" <- w99
            "TUBO" <- w96
            n152 = case shown="False" "Case Constant\n(See Context Help)" {
              selector: "Case Constant\n(See Context Help)" -> [_ w244]
              tunnel: w118 -> [w243 _]
              tunnel: [w242 _] -> w89
              tunnel: [w241 _] -> w120
              tunnel: [w240 w244] -> w119
              tunnel: [w239 _] -> w102
              frame False {
                n153 = call "Get Status Controlador.vi"("Controlador"=w243) -> ("Status"=w239:string, "Parametros"=w241:string, "Bits Status"=w242:bool[], "Erro comunicação"=w240:bool)
              }
              frame True {
              }
            }
            "AH_STAT" <- w102
            "RA" <- w89
            n154 = Equal?(x=w85, y="00") -> (x = y?=w83:bool)
            n155 = stacked-sequence {
              frame #0 {
                # "Verifica se exite o arquivo da trapeira"
                # "Lê do arquivo qual o estado atual da trapeira"
                n156 = String To Path(string="C:\\TCS\\LOG\\SHUTTER\\SHUTTER.TXT" ("pathLogFocoString")) -> (path=w124:path)
                n157 = call <vilib>:"Check if File or Folder Exists.vi"("path"=w124) -> ("file or folder exists?"=w122:bool, "dup path"=w121:path)  [unwired: 8 in, 1 out]
                n158 = case shown="True" w122 {
                  tunnel: w121 -> [_ w134]
                  frame False {
                    n159 = local write "StatShutterFile"(" " ("StatShutterFile")) -> ()
                  }
                  frame True {
                    n160 = Open/Create/Replace File(file path (use dialog)=w134, operation (0:open)=T6."open", access (0:read/write)=enum16{"read/write", "read-only", "write-only"}."read/write") -> (refnum out=w131:refnum<file>, error out=w126:errorcluster)  [unwired: 3 in, 1 out]
                    n161 = Read from Text File(file (use dialog)=w131, error in=w126) -> (text=w130:string)  [unwired: 2 in, 3 out]
                    n162 = Match Pattern(string=w130, regular expression="SHUTTER") -> (after substring=w128:string)  [unwired: 1 in, 3 out]
                    n163 = call <vilib>:"Trim Whitespace.vi"("string"=w128) -> ("trimmed string"=w127:string)  [unwired: 1 in]
                    n164 = case shown="\"OPENED\", Default" w127 {
                      selector: w127 -> [w135 w136]
                      frame "OPENED", Default {
                        "StatShutterFile" <- w135
                      }
                      frame "CLOSED" {
                        n165 = local write "StatShutterFile"(w136) -> ()
                      }
                    }
                  }
                }
              }
              frame #1 {
                n166 = local read "timeStatShutterAlert"() -> (w139:i32)
                n167 = Tick Count (ms)() -> (millisecond timer value=w141:u32)
                n168 = Add(x=w139, y=3000) -> (x+y=w140:i32)
                n169 = Greater Or Equal?(x=w141, y=w140) -> (x >= y?=w137:bool)
                n170 = case shown="True" w137 {
                  frame False {
                  }
                  frame True {
                    n171 = local read "StatShutterFile"() -> (w143:string)
                    n172 = property on="LedShutter" class="Bool (strict)"() -> ("BoolText.Text"=w144:string)  [unwired: 2 in, 2 out]
                    n173 = Not Equal?(x=w144, y=w143) -> (x != y?=w142:bool)
                    n174 = case shown="False" w142 {
                      frame True {
                        n175 = property on="StatShutterFile" class="Str"("Blinking"=TRUE) -> ()  [unwired: 2 in, 2 out]
                      }
                      frame False {
                        n176 = property on="StatShutterFile" class="Str"("Blinking"=FALSE) -> ()  [unwired: 2 in, 2 out]
                      }
                    }
                  }
                }
              }
              frame #2 {
                n177 = disable-structure shown="Disabled" {
                  frame Disabled {
                    n178 = local read "StatShutterFile"() -> (w148:string)
                    n179 = property on="LedShutter" class="Bool (strict)"() -> ("BoolText.Text"=w149:string)  [unwired: 2 in, 2 out]
                    n180 = Not Equal?(x=w149, y=w148) -> (x != y?=w147:bool)
                    n181 = case shown="True" w147 {
                      frame False {
                        n182 = property on="Setup, Pointing & Guiding" class="TabCtl (strict)"() -> ("Pages"=w151:refnum<vi>[])  [unwired: 2 in, 2 out]
                        n183 = Index Array(array=w151, index=6) -> (element=w152:refnum<vi>)
                        n184 = property class="Page"(reference=w152, "FG Color"=u32 12369084) -> ()  [unwired: 1 in, 2 out]
                      }
                      frame True {
                        n185 = property on="Setup, Pointing & Guiding" class="TabCtl (strict)"() -> ("Pages"=w159:refnum<vi>[])  [unwired: 2 in, 2 out]
                        n186 = Index Array(array=w159, index=6) -> (element=w158:refnum<vi>)
                        n187 = property class="Page"(reference=w158) -> ("FG Color"=w155:u32)  [unwired: 1 in, 2 out]
                        n188 = Equal?(x=w155, y=u32 16711680) -> (x = y?=w154:bool)
                        n189 = case shown="False" w154 {
                          frame False {
                            n190 = property on="Setup, Pointing & Guiding" class="TabCtl (strict)"() -> ("Pages"=w161:refnum<vi>[])  [unwired: 2 in, 2 out]
                            n191 = Index Array(array=w161, index=6) -> (element=w162:refnum<vi>)
                            n192 = property class="Page"(reference=w162, "FG Color"=u32 16711680) -> ()  [unwired: 1 in, 2 out]
                          }
                          frame True {
                            n193 = property on="Setup, Pointing & Guiding" class="TabCtl (strict)"() -> ("Pages"=w165:refnum<vi>[])  [unwired: 2 in, 2 out]
                            n194 = Index Array(array=w165, index=6) -> (element=w166:refnum<vi>)
                            n195 = property class="Page"(reference=w166, "FG Color"=u32 12369084) -> ()  [unwired: 1 in, 2 out]
                          }
                        }
                      }
                    }
                  }
                  frame Enabled {
                  }
                }
              }
            }
            n196 = case shown="True" w83 {
              frame False {
              }
              frame True {
                n197 = local read "Foco"() -> (w174:dbl)
                n198 = Number To Decimal String(number=w174) -> (decimal integer string=w173:string)  [unwired: 1 in]
                n199 = call "Log_Foco.vi"("command"=" ", "focValue"=w173, "pathLogFocoString"="C:\\TCS\\LOG\\FOCO\\") -> ()  [unwired: 6 in]
              }
            }
            n200 = Index Array(array=w96, index=3) -> (element=w94:bool)
            n201 = call "Testa_Comunicação.vi"("DEC"=w88, "RA"=w89) -> ()  [unwired: 10 in]
            n202 = case shown="True" w94 {
              tunnel: ["S" "M"] -> w93
              frame False {
              }
              frame True {
              }
            }
            n203 = global write "Global_Telescopio.vi" "MOTOR LIGADO"(w93) -> ()
            n204 = case shown="False" w119 {
              tunnel: w89 -> [w231 _]
              tunnel: w120 -> [w230 _]
              tunnel: [w228 _] -> w105
              frame False {
                # "Leitura Válida"
                n205 = call <vilib>:"Trim Whitespace.vi"("string"=w230) -> ("trimmed string"=w228:string)  [unwired: 1 in]
                n206 = call "hms_rad.vi"("True = hora"=TRUE, "Texto Graus"=w228) -> ("radianos"=w225:dbl)  [unwired: 3 in]
                n207 = global write "Global_Telescopio.vi" "StatusAH"(w231) -> ()
                n208 = global read "Global_Telescopio.vi" "PosAH"() -> (w227:dbl)
                n209 = Equal?(x=w227, y=w225) -> (x = y?=w226:bool)
                n210 = case shown="False" w226 {
                  tunnel: w225 -> [w234 _]
                  frame False {
                    w233 = 0 ("CR AH")
                    n211 = local write "CR AH"(w233) -> ()
                    n212 = local write "CR AH UTILS"(w233) -> ()
                    n213 = global write "Global_Telescopio.vi" "PosAH"(w234) -> ()
                    "PosAH" <- w234
                    "Flag ativo AH" <- TRUE ("Flag ativo AH")
                  }
                  frame True {
                    n214 = local read "CR AH UTILS"() -> (w236:i32)
                    n215 = Increment(x=w236) -> (x+1=w235:i32)
                    n216 = local read "CR AH"() -> (w237:i32)
                    n217 = Increment(x=w237) -> (x+1=w238:i32)
                    n218 = local write "CR AH UTILS"(w235) -> ()
                    n219 = local write "CR AH"(w238) -> ()
                  }
                }
              }
              frame True {
                # "Erro na Leitura"
              }
            }
            "AH_ENC" <- w105
            n220 = case shown="False" w116 {
              tunnel: w117 -> [w216 _]
              tunnel: w88 -> [w215 _]
              tunnel: [w214 _] -> w104
              frame False {
                # "Leitura Válida"
                n221 = call <vilib>:"Trim Whitespace.vi"("string"=w216) -> ("trimmed string"=w214:string)  [unwired: 1 in]
                n222 = call "hms_rad.vi"("True = hora"=FALSE, "Texto Graus"=w214) -> ("radianos"=w211:dbl)  [unwired: 3 in]
                n223 = global write "Global_Telescopio.vi" "StatusDEC"(w215) -> ()
                n224 = global read "Global_Telescopio.vi" "PosDEC"() -> (w213:dbl)
                n225 = Equal?(x=w213, y=w211) -> (x = y?=w212:bool)
                n226 = case shown="False" w212 {
                  tunnel: w211 -> [w220 _]
                  frame False {
                    w219 = 0 ("CR DEC")
                    n227 = local write "CR DEC UTILS"(w219) -> ()
                    n228 = local write "CR DEC"(w219) -> ()
                    n229 = global write "Global_Telescopio.vi" "PosDEC"(w220) -> ()
                    "PosDEC" <- w220
                    "Flag ativo DEC" <- TRUE ("Flag ativo DEC")
                  }
                  frame True {
                    n230 = local read "CR DEC"() -> (w224:i32)
                    n231 = local read "CR DEC UTILS"() -> (w222:i32)
                    n232 = Increment(x=w222) -> (x+1=w221:i32)
                    n233 = Increment(x=w224) -> (x+1=w223:i32)
                    n234 = local write "CR DEC UTILS"(w221) -> ()
                    n235 = local write "CR DEC"(w223) -> ()
                  }
                }
              }
              frame True {
                # "Erro na Leitura"
              }
            }
            "DEC_ENC" <- w104
            n236 = case shown="False" w113 {
              tunnel: w98 -> [w198 _]
              tunnel: w112 -> [w197 _]
              tunnel: [w195 _] -> w103
              frame False {
                # "Leitura Válida"
                n237 = call <vilib>:"Trim Whitespace.vi"("string"=w197) -> ("trimmed string"=w195:string)  [unwired: 1 in]
                n238 = Decimal String To Number(string=w195) -> (number=w196:i32)  [unwired: 2 in, 1 out]
                n239 = global write "Global_Telescopio.vi" "StatusCUP"(w198) -> ()
                n240 = global write "Global_Telescopio.vi" "PosCUP"(w196) -> ()
              }
              frame True {
                # "Erro na Leitura"
              }
            }
            "DOMO_ENC" <- w103
            n241 = case shown="False" w107 {
              tunnel: w96 -> [w187 _]
              tunnel: w108 -> [w182 _]
              frame False {
                # "Leitura Válida"
                n242 = call <vilib>:"Trim Whitespace.vi"("string"=w182) -> ("trimmed string"=w186:string)  [unwired: 1 in]
                n243 = Decimal String To Number(string=w186) -> (number=w185:i32)  [unwired: 2 in, 1 out]
                n244 = global write "Global_Telescopio.vi" "StatusTUBO"(w187) -> ()
                n245 = global write "Global_Telescopio.vi" "PosFOCO"(w185) -> ()
                n246 = String Subset(string=w182, offset (0)=10, length (rest)=1 ("length (rest)")) -> (substring=→"EspAtual":string)
                n247 = Number To Decimal String(number=w185) -> (decimal integer string=w180:string)  [unwired: 1 in]
                "FOCO_ENC" <- w180
                n248 = Decimal String To Number(string=w180) -> (number=w178:i32)  [unwired: 2 in, 1 out]
                n249 = Greater Than 0?(x=w178) -> (x > 0?=w179:bool)
                n250 = case shown="True" w179 {
                  tunnel: w178 -> [_ w188]
                  frame False {
                  }
                  frame True {
                    n251 = global write "Global_Telescopio.vi" "Foco"(w188) -> ()
                  }
                }
              }
              frame True {
                # "Erro na Leitura"
              }
            }
            n252 = local read "shutterTimeOld"() -> (w82:i32)
            n253 = local read "sendCommandShutter"() -> (w77:bool)
            n254 = Tick Count (ms)() -> (millisecond timer value=w80:u32)
            n255 = Add(x=w82, y=40000) -> (x+y=w79:i32)
            n256 = Greater Or Equal?(x=w80, y=w79) -> (x >= y?=w78:bool)
            n257 = And(x=w78, y=w77) -> (x .and. y?=w76:bool)
            n258 = call "Sideral_Time.vi"("Fuso"=-3.0) -> ("TU"=→"UT":string, "Sideral Time"=w109:dbl)  [unwired: 2 in, 1 out]
            n259 = local read "LedPointing"() -> (w91:bool)
            n260 = case shown="True" w76 {
              frame False {
              }
              frame True {
                w168 = u16 4 items=["ZERO", "AH", "DEC", "TUBO", "CUP"] ("Controlador")
                # "Envia o comando para o controlador\nda cupula, após 40 segundos"
                n261 = local write "sendCommandShutter"(FALSE ("writeShutterLog")) -> ()
                n262 = call "Monta Comando.vi"("Comando"="PARAR", "Dispositivo"="TRAPEIRA" ("Comando"), "Controlador"=w168) -> ()  [unwired: 4 in, 3 out]
              }
            }
            n263 = local read "MOVING"() -> (w92:bool)
            n264 = global write "Global_Telescopio.vi" "Sideral Time"(w109) -> ()
            n265 = Or(x=w91, y=w92) -> (x .or. y?=w90:bool)
            n266 = shared-variable "My Computer\\Shared_160.lvlib\\Beep"(w90) -> ()  [unwired: 1 in, 1 out]
          }
          frame #1 {
            w258 = u16 9 items=["Alarme", "Atencao", "Erro", "Ocupado", "Protecao", "Embreagem", "Tracking", "Var. Track", "Rápido", "Ligeiro", "Médio", "Lento", "Em movimento", ""] ("NomeStatus")
            w259 = u16 9 items=["Alarme", "Atencao", "Erro", "Ocupado", "Protecao", "Embreagem", "Tracking", "Var. Track", "Rápido", "Ligeiro", "Médio", "Lento", "Em movimento", ""] ("NomeStatus")
            w262 = u16 8 items=["Alarme", "Atencao", "Erro", "Ocupado", "Protecao", "Embreagem", "Tracking", "Var. Track", "Rápido", "Ligeiro", "Médio", "Lento", "Em movimento", ""] ("NomeStatus")
            w263 = u16 8 items=["Alarme", "Atencao", "Erro", "Ocupado", "Protecao", "Embreagem", "Tracking", "Var. Track", "Rápido", "Ligeiro", "Médio", "Lento", "Em movimento", ""] ("NomeStatus")
            w269 = 6.283185307179586
            # "Desabilita botões \"Precess\" e \"Clear\"\ndurante o apontamento"
